vi "Num2Str_TrailingZero.vi"(11 "Numeric Control":u32) -> (3 "format string":string)   [LabVIEW 2020]
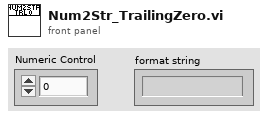
[diagram p1: front panel]
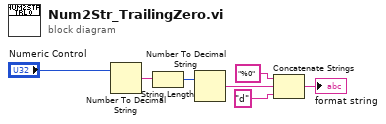
[diagram p0: block diagram]
diagram:
  n1 = Number To Decimal String(number="Numeric Control") -> (decimal integer string=w7:string)  [unwired: 1 in]
  n2 = String Length(string=w7) -> (length=w6:i32)
  n3 = Number To Decimal String(number=w6) -> (decimal integer string=w4:string)  [unwired: 1 in]
  n4 = Concatenate Strings("%0" ("format string"), w4, "d" ("format string")) -> (→"format string":string)
